vi "Create Name Msg Refs.vi"(6 "Name Msg":string, 8 "error in":errorcluster, 9 "Name Library File Path":path, 10 "Active Project":refnum<vi>) -> (0 "error out":errorcluster, 2 "Name Msg Refs":T1)   [LabVIEW 2025, in "_Msg Rescript.lvlib" / "_Msg Rescript.lvclass"]
uses:
  _Msg Rescript.lvclass
  Name Msg Refs.ctl
  <vilib>/Utility/traverseref.llb/TRef TravTarget.ctl
  _Msg Rescript.lvclass/_Msg Rescript.ctl
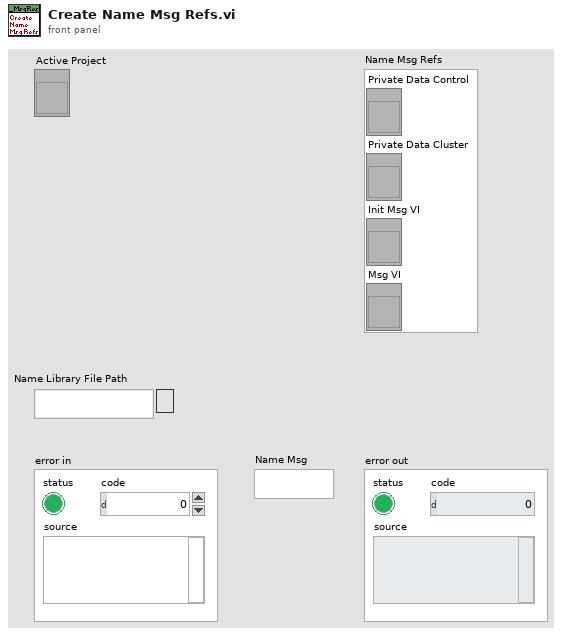
[diagram p1: front panel]
types:
  T1 = typedef "_Msg Rescript.lvlib/_Msg Rescript.lvclass/Name Msg Refs.ctl" = cluster{"Private Data Control":refnum<vi>, "Private Data Cluster":refnum<vi>, "Init Msg VI":refnum<vi>, "Msg VI":refnum<vi>}
  T2 = typedef "TRef TravTarget.ctl" = enum16{"FP", "BD", "Other"}
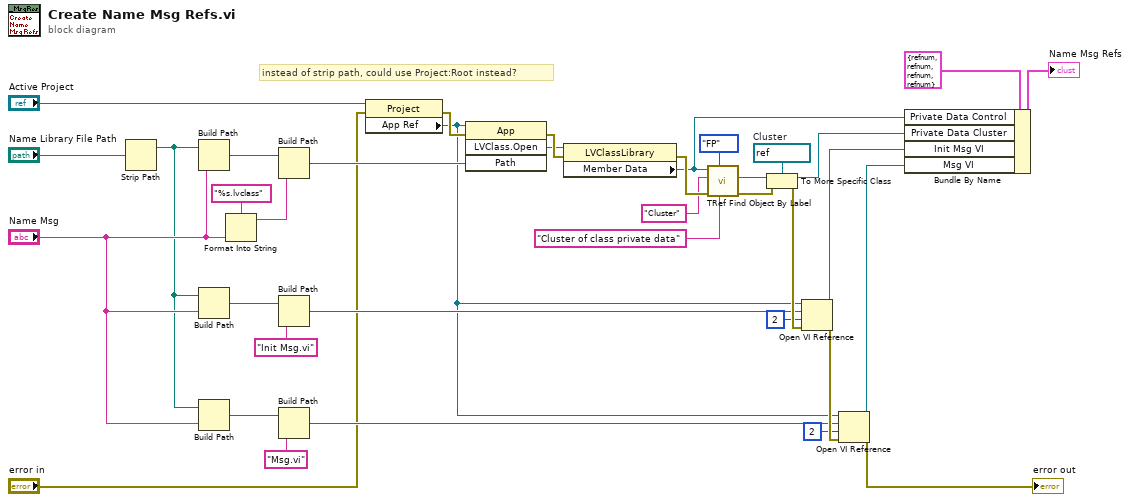
[diagram p0: block diagram]
diagram:
  w31 = refnum<vi> refnum  # Cluster
  # "instead of strip path, could use Project:Root instead?"
  n1 = Strip Path(path="Name Library File Path") -> (stripped path=w10:path)  [unwired: 1 out]
  n2 = Build Path(base path=w10, name or relative path="Name Msg") -> (appended path=w25:path)
  n3 = Build Path(base path=w10, name or relative path="Name Msg") -> (appended path=w21:path)
  n4 = Build Path(base path=w10, name or relative path="Name Msg") -> (appended path=w20:path)
  n5 = Format Into String(format string="%s.lvclass", "Name Msg") -> (resulting string=w23:string)  [unwired: 2 in, 1 out]
  n6 = Build Path(base path=w25, name or relative path=w23) -> (appended path=w24:path)
  n7 = Build Path(base path=w21, name or relative path="Init Msg.vi" ("format string")) -> (appended path=w17:path)
  n8 = Build Path(base path=w20, name or relative path="Msg.vi" ("format string")) -> (appended path=w16:path)
  n9 = property class="Project"(reference="Active Project", error in="error in") -> (error out=w35:errorcluster, "App Ref"=w9:refnum<vi>)  [unwired: 1 out]
  n10 = invoke class="App" method="LVClass.Open"(reference=w9, error in=w35, "Path"=w24) -> (error out=w33:errorcluster, "LVClass.Open"=w26:refnum<vi>)  [unwired: 1 in, 2 out]
  n11 = property class="LVClassLibrary"(reference=w26, error in=w33) -> (error out=w37:errorcluster, "Member Data"=w6:refnum<vi>)  [unwired: 1 out]
  n12 = call <vilib>:"TRef Find Object By Label.vi"("Label"="Cluster of class private data" ("Class Name"), "Traverse Target"=TRef_TravTarget."FP", "error in (no error)"=w37, "Class Name"="Cluster", "VI Ref"=w6) -> ("error out"=w32:errorcluster, "Found Obj Ref"=w30:refnum<vi>)  [unwired: 3 in, 2 out]
  n13 = To More Specific Class(target class=w31, reference=w30, error in=w32) -> (specific class reference=w5:refnum<vi>, error out=w34:errorcluster)
  n14 = Open VI Reference(application reference (local)=w9, vi path=w17, options=2, error in (no error)=w34) -> (vi reference=w4:refnum<vi>, error out=w36:errorcluster)  [unwired: 2 in]
  n15 = Open VI Reference(application reference (local)=w9, vi path=w16, options=2, error in (no error)=w36) -> (vi reference=w3:refnum<vi>, error out=→"error out":errorcluster)  [unwired: 2 in]
  n16 = Bundle By Name(cluster=T1 {"Private Data Control"=refnum, "Private Data Cluster"=refnum, "Init Msg VI"=refnum, "Msg VI"=refnum} ("Name Msg Refs"), "Private Data Control"=w6, "Private Data Cluster"=w5, "Init Msg VI"=w4, "Msg VI"=w3) -> (→"Name Msg Refs":T1)
